vi "Store Subpanel References.vi"(8 "error in (no error)":errorcluster, 10 "Subpanel References":refnum<vi>[](array[refnum]), 11 "GUI Container in":refnum<class "GUI Container.lvclass">) -> (0 "error out":errorcluster, 2 "Sub Panel Names":string[](array[string]), 3 "GUI Container out":refnum<class "GUI Container.lvclass">)   [LabVIEW 2023, in "GUI Views.lvlib" / "GUI Container.lvclass"]
doc: "This method is used within the \"Actor Core.vi\" of the concrete \"GUI Container\" to store the references of the subpanels present in its front panel and that we want to use as containers."
uses:
  GUI Container.lvclass
  GUI Container.lvclass/GUI Container.ctl
  typedefs/Subpanel Status.ctl
  <userlib>/_OpenG.lib/error/error.llb/openg_error.lvlib
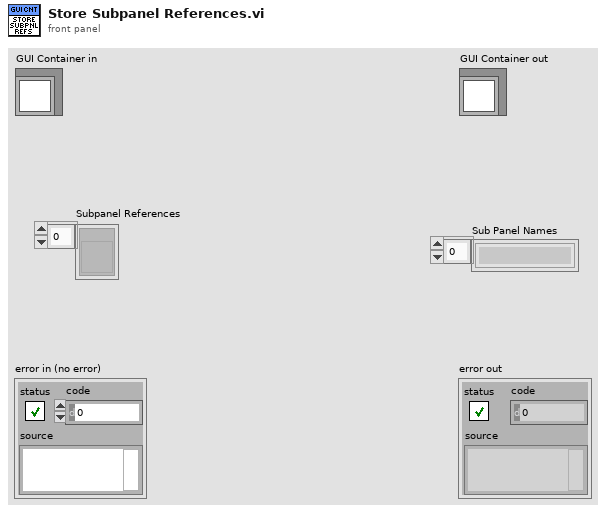
[diagram p1: front panel]
types:
  T1 = typedef "GUI Views.lvlib/GUI Container.lvclass/Subpanel Status.ctl" = cluster{"Subpanel Ref":refnum<vi>, "Inserted View":string, "Inserted View Hierarchy Level":i32}
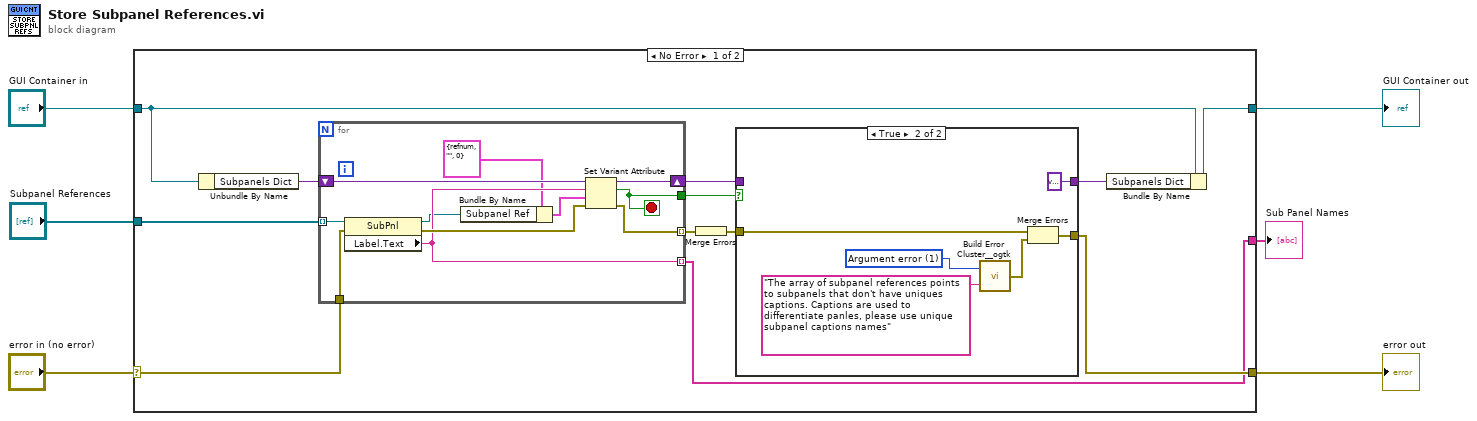
[diagram p0: block diagram]
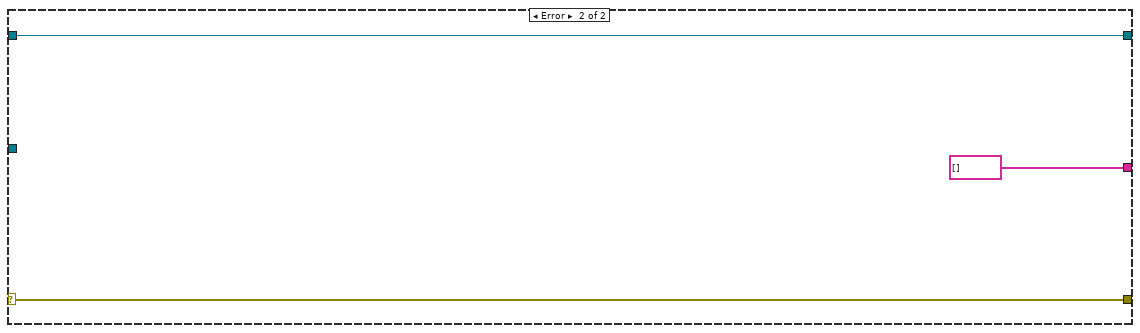
[diagram p3: hidden frame]
diagram:
  n1 = case shown="No Error" "error in (no error)" {
    selector: "error in (no error)" -> [w15 w40]
    tunnel: [w11 w40] -> w5
    tunnel: [w9 w39] -> w3
    tunnel: "GUI Container in" -> [w17 w39]
    tunnel: "Subpanel References" -> [w18 _]
    tunnel: [w7 string[] []] -> w1
    frame No Error {
      n2 = Unbundle By Name(w17) -> ("Subpanels Dict"=w16:variant)
      n3 = for {
        tunnel: w18 -> [w36] mode=indexing
        tunnel: w15 -> [w35]
        tunnel: [w33] -> w14 mode=indexing
        shift-right: [w32] -> w10
        shift-left: w16 -> [w37]
        tunnel: [w31] -> w13
        tunnel: [w30] -> w7 mode=indexing
        stop <- w31 stop-if-true
        n4 = property class="SubPnl"(reference=w36, error in=w35) -> (reference out=w28:refnum<vi>, error out=w34:errorcluster, "Label.Text"=w30:string)
        n5 = Bundle By Name(cluster=T1 {"Subpanel Ref"=refnum, "Inserted View"="", "Inserted View Hierarchy Level"=0} ("Subpanel Status"), "Subpanel Ref"=w28) -> (w27:T1)
        n6 = Set Variant Attribute(Variant=w37, name=w30, value=w27, error in=w34) -> (Variant out=w32:variant, replaced=w31:bool, error out=w33:errorcluster)
      }
      n7 = Merge Errors(w14) -> (w12:errorcluster)
      n8 = case shown="True" w13 {
        tunnel: w12 -> [w20 w24]
        tunnel: [w20 w22] -> w11
        tunnel: w10 -> [w19 _]
        tunnel: [w19 variant ("Subpanels")] -> w8
        frame False {
        }
        frame True {
          w26 = 1 items=["No error", "Argument error", "Memory is full", "Out of zone", "End of file", "File already open", "Generic file I/O error", "File not found", "File permission error", "Disk is full", "Duplicate path", "Too many files open", "System feature not enabled", "Resource file not found", "Cannot add resource", "Resource not found", "Image not found", "Image memory error", "Pen does not exist", "Config type invalid", "Config token not found", "Config parse error", "Config memory error", "Bad external code format", "Bad external code offset", "External code not present", "Null window", "Destroy window error", "Null menu", "Print aborted", "Bad print record", "Print driver error", "Windows error during printing", "Memory error during printing", "Print dialog error", "Generic print error", "Invalid device refnum", "Device not found", "Device parameter error", "Device unit error", "Cannot open device", "Device call aborted", "Generic error", "Cancelled by user", "Object ID too low", "Object ID too high", "Object not in heap", "Unknown heap", "Unknown object (invalid DefProc)", "Unknown object (DefProc not in table)", "Message out of range", "Invalid (null) method", "Unknown message", "Manager call not supported", "Bad address", "Network operation in progress", "Network operation timed out", "Connection is busy", "Network attribute not supported", "Network error", "Address in use", "System out of memory", "Connection aborted", "Connection refused", "Not connected", "Already connected", "Connection closed", "Initialization error (interapplication manager)", "Bad occurrence", "Wait on unbound occurrence handler", "Occurrence queue overflow", "Datalog type conflict", "Unused", "Unrecognized type (interapplication manager)", "Memory corrupt", "Failed to make temporary DLL", "Old CIN version", "Drag socket not found", "Failed to load drop-object", "Failed to register OLE object", "Failed to release OLE object", "Format specifier type mismatch", "Unknown format specifier", "Too few format specifiers", "Too many format specifiers", "Scan failed", "Newer CIN version", "Error converting to variant", "Runtime menu error", "Password tampered", "Variant attribute not found", "Incompatible variant data type", "Event data is not available", "Event Store is not present", "Occurrence is not found", "Event Queue is not created", "Event info is not available", "Refnum passed is NULL", "Error retrieving Class GUID", "Error retrieving CoClass GUID", "Error retrieving TypeLib GUID.", "Bad built application magic bytes.", "Specific driver is different from the specific driver associated with the Logical Name.", "There is no session opened to the class driver.", "Max Error", "MAX - Error with config objects", "MAX - Error loading configuration", "MAX - Group not supported"]
          n9 = call <userlib>:"Build Error Cluster__ogtk.vi"("String to Prepend to source (\"\")"="The array of subpanel references points to subpanels that don't have uniques captions. Captions are used to differentiate panles, please use unique subpanel captions names" ("String to Prepend to source (\"\")"), "code"=w26) -> ("error out"=w23:errorcluster)
          n10 = Merge Errors(w24, w23) -> (w22:errorcluster)
        }
      }
      n11 = Bundle By Name(cluster=w17, "Subpanels Dict"=w8) -> (w9:refnum<class "GUI Container.lvclass">)
    }
    frame Error {
    }
  }
  "error out" <- w5
  "GUI Container out" <- w3
  "Sub Panel Names" <- w1
